vi "DCC_get_eeprom_data.vi"(8 "Error In":errorcluster, 10 "Module No":i16, 11 "DLL Path":path) -> (0 "Error Out":errorcluster, 2 "Module No":i16, 3 "DLL Path":path, 4 "EEPROM Data":T1)   [LabVIEW 2019]
doc: "The function \"DDC_get_eeprom_data\"will be called from this VI to get the EEPROM data stored in the memory of the card specified by the module number.\nThe module number has to be in the range of 0 until 7 in integer steps.\n\nOctober 2018\nFrank Quadt & Stefan Smietana\ninfo@becker-hickl.com"
uses:
  DCC_Controls/DCC_EEP_Data_Cluster.ctl
panel:
  # "(c) 2021 Becker & Hickl GmbH\n     All Rights Reserved."
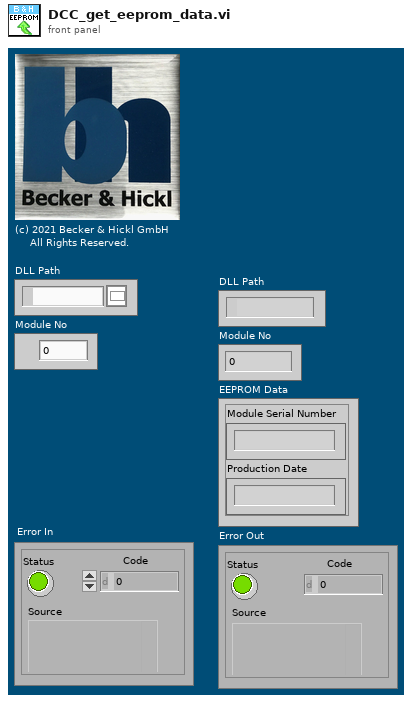
[diagram p1: front panel]
types:
  T1 = typedef "DCC_EEP_Data_Cluster.ctl" = cluster{"Module Serial Number":string, "Production Date":string}
  T2 = cluster{"[0]":u8, "[1]":u8, "[2]":u8, "[3]":u8, "[4]":u8, "[5]":u8, "[6]":u8, "[7]":u8, "[8]":u8}
  T3 = cluster{cluster{"[0]":u8, "[1]":u8, "[2]":u8, "[3]":u8, "[4]":u8, "[5]":u8, "[6]":u8, "[7]":u8, "[8]":u8}, cluster{"[0]":u8, "[1]":u8, "[2]":u8, "[3]":u8, "[4]":u8, "[5]":u8, "[6]":u8, "[7]":u8, "[8]":u8}}
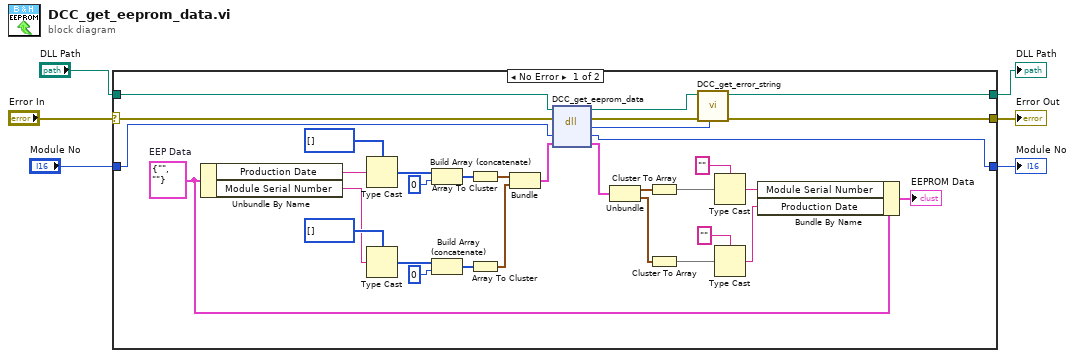
[diagram p0: block diagram]
diagram:
  n1 = case shown="No Error" "Error In" {
    selector: "Error In" -> [w39 w41]
    tunnel: [w31 w41] -> w5
    tunnel: [w34 w40] -> w4
    tunnel: "DLL Path" -> [w37 w40]
    tunnel: "Module No" -> [w36 w42]
    tunnel: [w35 w42] -> w1
    frame No Error {
      w7 = T1 {"Module Serial Number"="", "Production Date"=""}  # EEP Data
      n2 = Unbundle By Name(w7) -> ("Production Date"=w25:string, "Module Serial Number"=w20:string)
      n3 = Type Cast(type=u8[] [], x=w25) -> (*(type *) &x=w27:u8[])
      n4 = Type Cast(type=u8[] [], x=w20) -> (*(type *) &x=w23:u8[])
      n5 = Build Array (concatenate)(w27, u8 0) -> (w29:u8[])
      n6 = Build Array (concatenate)(w23, u8 0) -> (w21:u8[])
      n7 = Array To Cluster(array=w29) -> (cluster=w30:T2)
      n8 = Array To Cluster(array=w21) -> (cluster=w19:T2)
      n9 = Bundle(w30, w19) -> (w18:T3)  [unwired: 1 in]
      n10 = dll-call lib="C:/Program Files/BH/DCC/DLL/dcc32.dll" fn="DCC_get_eeprom_data"(path in=w37, error in=w39, "ModuleNo"=w36, "EepromData"=w18) -> (path out=w38:path, error out=w33:errorcluster, "return type"=w32:i16, "ModuleNo"=w35:i16, "EepromData"=w17:T3)  [unwired: 1 in]
      n11 = Unbundle(w17) -> (w16:T2, w15:T2)
      n12 = Cluster To Array(cluster=w16) -> (array=w8:u8[])
      n13 = Cluster To Array(cluster=w15) -> (array=w9:u8[])
      n14 = call "DCC_get_error_string.vi"("Error ID"=w32, "Error In"=w33, "DLL Path"=w38) -> ("Error Out"=w31:errorcluster, "DLL Path"=w34:path)  [unwired: 6 in, 1 out]
      n15 = Type Cast(type="", x=w8) -> (*(type *) &x=w11:string)
      n16 = Type Cast(type="", x=w9) -> (*(type *) &x=w10:string)
      n17 = Bundle By Name(cluster=w7, "Module Serial Number"=w11, "Production Date"=w10) -> (→"EEPROM Data":T1)
    }
    frame Error {
    }
  }
  "Error Out" <- w5
  "DLL Path" <- w4
  "Module No" <- w1
